vi "WhereForebrainPerception.vi"(2 "Where? Midbrain":T1) -> (1 "SimPitchRoll":dbl, 5 "Where? Forebrain":T1, 6 "(xr,yr)":cluster{"X":dbl, "Y":dbl}, 7 "Direction":dbl)   [LabVIEW 2012]
doc: "This SubVI takes clean Where sense data from the Midbrain and layers perception onto it to be passed to the THINK processes in the Forebrain\n\nT=time\nxr=horizontal coordiante\nyr=vertical coordinate"
panel:
  # "This SubVI adds \nperception onto the\nWhere data comming\nfrom the Midbrain"
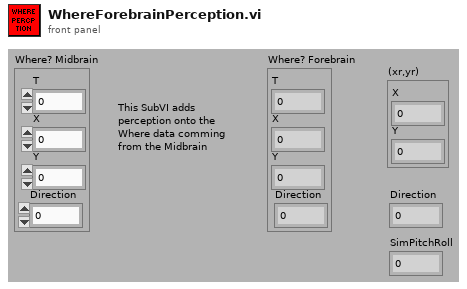
[diagram p1: front panel]
types:
  T1 = cluster{"T":dbl, "X":dbl, "Y":dbl, "Direction":dbl}
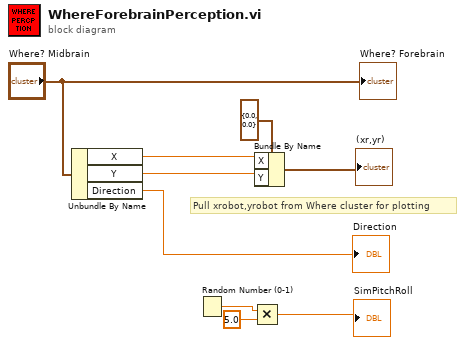
[diagram p0: block diagram]
diagram:
  # "Pull xrobot,yrobot from Where cluster for plotting"
  n1 = Unbundle By Name("Where? Midbrain") -> ("X"=w7:dbl, "Y"=w6:dbl, "Direction"=→"Direction":dbl)
  n2 = Random Number (0-1)() -> (number: 0 to 1=w3:dbl)
  n3 = Multiply(x=w3, y=5.0) -> (x*y=→"SimPitchRoll":dbl)
  n4 = Bundle By Name(cluster=cluster{"X":dbl, "Y":dbl} {"X"=0.0, "Y"=0.0} ("(xr,yr)"), "X"=w7, "Y"=w6) -> (→"(xr,yr)":cluster{"X":dbl, "Y":dbl})
  "Where? Forebrain" <- "Where? Midbrain"
